vi "Data Storage - Get Element Count (B256).vi"(0 "# of bits":u64, 2 "reset":bool, 5 "read enable":bool, 7 "bit counter enable":bool) -> (4 "memory size":u32, 6 "bit count":u16)   [LabVIEW 2018, in "Streaming FPGA.lvlib"]
doc: "Data Storage memory mode element counter for B256 elements.\n \nThe <B>memory size</B> output returns the number of B256 elements required to store <B># of bits</B> booleans. Set the <B>read enable</B> input to true in each clock cycle when the memory is read and the <B>bit count</B> output returns the number of valid boolean elements read from the memory in the current cycle, assuming that following a reset the memory read starts from the first element, each read operation reads 256 elements and after reading the memory <B>memory size</B> number of times the read continues from the first element. If the <B>bit counter enable</B> input is false, then the <B>bit count</B> output is set to 256."
uses:
  Streaming FPGA.lvlib
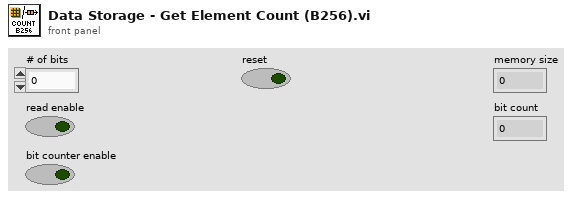
[diagram p1: front panel]
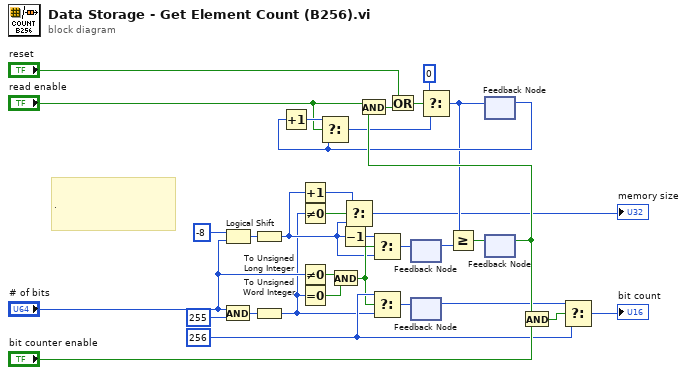
[diagram p0: block diagram]
diagram:
  w13 = u16 256 ("f")
  # "Each DRAM memory element is an array of 256 booleans."
  # "."
  # "."
  n1 = Logical Shift(y=i16 -8, x="# of bits") -> (x << y=w6:u64)
  n2 = And(x="# of bits", y=u64 255) -> (x .and. y?=w2:u64)
  n3 = To Unsigned Long Integer(number=w6) -> (unsigned 32bit integer=w3:u32)
  n4 = To Unsigned Word Integer(number=w2) -> (unsigned 16bit integer=w1:u16)
  n5 = Increment(x=w3) -> (x+1=w7:u32)
  n6 = Not Equal To 0?(x=w1) -> (x != 0?=w8:bool)
  n7 = Not Equal To 0?(x="# of bits") -> (x != 0?=w9:bool)
  n8 = Equal To 0?(x=w1) -> (x = 0?=w12:bool)
  n9 = And(x=w9, y=w12) -> (x .and. y?=w11:bool)
  n10 = Decrement(x=w3) -> (x-1=w16:u32)
  n11 = Select(t=w7, s=w8, f=w3) -> (s? t:f=→"memory size":u32)
  n12 = Select(t=w16, s=w11, f=w3) -> (s? t:f=w15:u32)
  n13 = Select(t=w13, s=w11, f=w1) -> (s? t:f=w14:u16)
  n14 = feedback #1() -> (w22:u32)  [unwired: 1 in]
  n15 = feedback-in #1(w15) -> ()
  n16 = feedback #2() -> (w20:u16)  [unwired: 1 in]
  n17 = feedback-in #2(w14) -> ()
  n18 = feedback #3() -> (w30:u32)  [unwired: 1 in]
  n19 = Increment(x=w30) -> (x+1=w29:u32)
  n20 = Select(t=w29, s="read enable", f=w30) -> (s? t:f=w27:u32)
  n21 = feedback #4() -> (w33:bool)  [unwired: 1 in]
  n22 = And(x="read enable", y=w33) -> (x .and. y?=w24:bool)
  n23 = Or(x="reset", y=w24) -> (x .or. y?=w28:bool)
  n24 = Select(t=u32 0, s=w28, f=w27) -> (s? t:f=w23:u32)
  n25 = Greater Or Equal?(x=w23, y=w22) -> (x >= y?=w26:bool)
  n26 = feedback-in #3(w23) -> ()
  n27 = feedback-in #4(w26) -> ()
  n28 = And(x=w33, y="bit counter enable") -> (x .and. y?=w4:bool)
  n29 = Select(t=w20, s=w4, f=w13) -> (s? t:f=→"bit count":u16)
